vi "initialize Imaq images and update cvt table.vi"(8 "error in (no error)":errorcluster) -> (0 "error out":errorcluster, 2 "spotfieldImage Out":T1, 3 "image out":T1)   [LabVIEW 2020]
uses:
  <vilib>/vision/Image Controls.llb/IMAQ Image.ctl
  shared/CompressAndUpdate(Poly)/CompressAndUpdate(IMAQ Image).vi
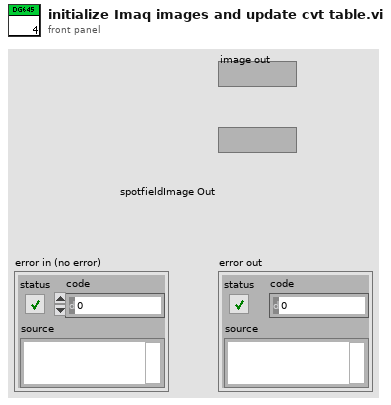
[diagram p1: front panel]
types:
  T1 = typedef "IMAQ Image.ctl" = refnum<image>
  T2 = typedef "Image Type" = u32
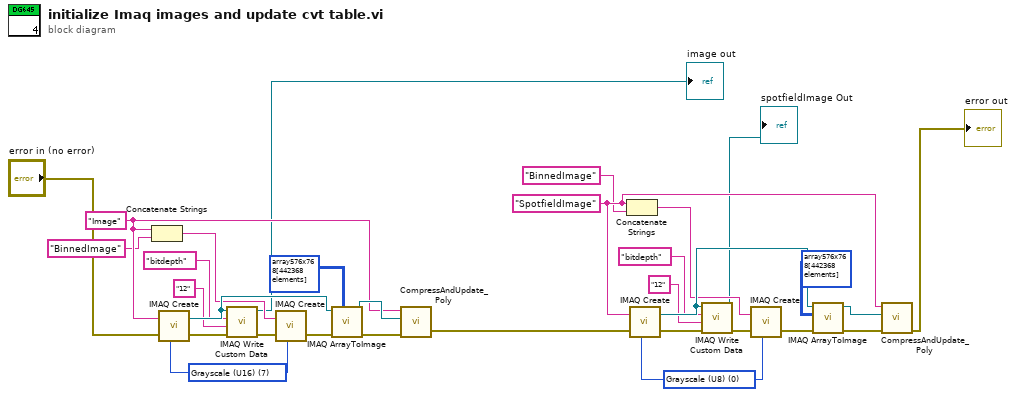
[diagram p0: block diagram]
diagram:
  w18 = "Image" ("string")
  w28 = "SpotfieldImage" ("Image Name")
  w14 = T2 0 items=["Grayscale (U8)", "Grayscale (I16)", "Grayscale (SGL)", "Complex (CSG)", "RGB (U32)", "HSL (U32)", "RGB (U64)", "Grayscale (U16)"] ("Image Type")
  w7 = T2 7 items=["Grayscale (U8)", "Grayscale (I16)", "Grayscale (SGL)", "Complex (CSG)", "RGB (U32)", "HSL (U32)", "RGB (U64)", "Grayscale (U16)"] ("Image Type")
  n1 = Concatenate Strings(w18, "BinnedImage" ("command or variable name")) -> (w17:string)
  n2 = call "IMAQ Create"("Image Name"=w18, "Image Type"=w7, "error in (no error)"="error in (no error)") -> ("New Image"=w20:T1, "error out"=w5:errorcluster)  [unwired: 2 in]
  n3 = call "IMAQ Write Custom Data"("error in (no error)"=w5, "Custom Data In"="12", "Key"="bitdepth", "Image"=w20) -> ("error out"=w6:errorcluster, "Image Out"=→"image out":T1)  [unwired: 6 in]
  n4 = call "IMAQ Create"("Image Name"=w17, "Image Type"=w7, "error in (no error)"=w6) -> ("error out"=w24:errorcluster)  [unwired: 2 in, 1 out]
  n5 = call "IMAQ ArrayToImage"("Image Pixels (U16)"=u8[][] array576x768[442368 elements] ("output array"), "error in (no error)"=w24, "Image"=w20) -> ("error out"=w22:errorcluster, "Image Out"=w27:T1)  [unwired: 7 in]
  n6 = call-poly "CompressAndUpdate_Poly.vi"("error in"=w22, "IMAQ Image"=w27, "command or variable name"=w18) -> ("error out"=w25:errorcluster)  [unwired: 8 in]
  n7 = Concatenate Strings(w28, "BinnedImage" ("command or variable name")) -> (w13:string)
  n8 = call "IMAQ Create"("Image Name"=w28, "Image Type"=w14, "error in (no error)"=w25) -> ("New Image"=w21:T1, "error out"=w11:errorcluster)  [unwired: 2 in]
  n9 = call "IMAQ Write Custom Data"("error in (no error)"=w11, "Custom Data In"="12", "Key"="bitdepth", "Image"=w21) -> ("error out"=w15:errorcluster, "Image Out"=→"spotfieldImage Out":T1)  [unwired: 6 in]
  n10 = call "IMAQ Create"("Image Name"=w13, "Image Type"=w14, "error in (no error)"=w15) -> ("error out"=w26:errorcluster)  [unwired: 2 in, 1 out]
  n11 = call "IMAQ ArrayToImage"("error in (no error)"=w26, "Image Pixels (U8)"=u8[][] array576x768[442368 elements] ("output array"), "Image"=w21) -> ("error out"=w31:errorcluster, "Image Out"=w30:T1)  [unwired: 7 in]
  n12 = call-poly "CompressAndUpdate_Poly.vi"("error in"=w31, "IMAQ Image"=w30, "command or variable name"=w28) -> ("error out"=→"error out":errorcluster)  [unwired: 8 in]
